vi "GCSArray_intersection.vi"(0 "Input keyword array":string[](array[string]), 1 "Available keyword array":string[](array[string]), 5 "error in (no error)":errorcluster) -> (14 "Intersection indices":i32[](array[numeric]), 19 "error out":errorcluster)   [LabVIEW 2020]
doc: "Find Intersection indices of the Input array in the Key array. The Key array acts as the master, where each element of Input array is searched. Only when equal elements are found the corresponding Input array index is added to the Intersection indices array."
panel:
  # "Find differences between two keyword arrays. Each entry of the\n'Input keyword array' is checked against any element stored in\n'Available keyword array' which acts as the master. Everytime\nan element was found its index of 'Input keyword array' is\nappended in the 'Intersection indices' list."
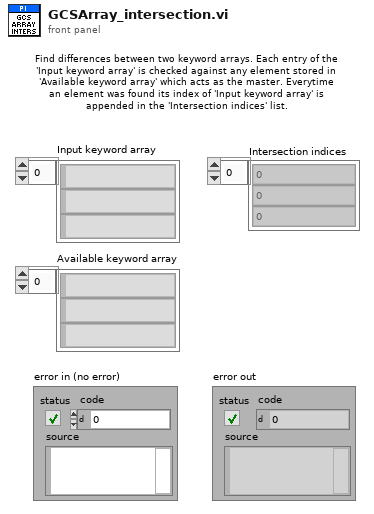
[diagram p1: front panel]
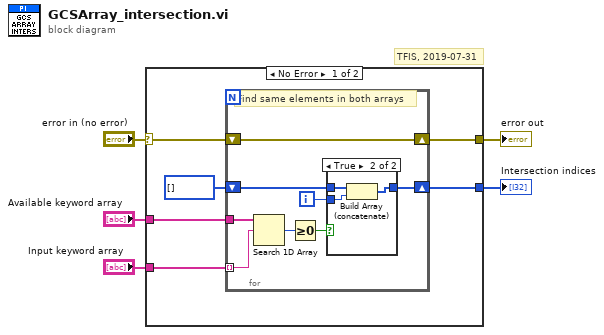
[diagram p0: block diagram]
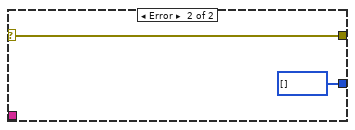
[diagram p3: hidden frame]
diagram:
  # "TFIS, 2019-07-31"
  n1 = case shown="No Error" "error in (no error)" {
    selector: "error in (no error)" -> [w11 w25]
    tunnel: [w10 w25] -> w4
    tunnel: [w9 i32[] []] -> w3
    tunnel: "Input keyword array" -> [w8 _]
    tunnel: "Available keyword array" -> [w7 _]
    frame No Error {
      n2 = for {
        tunnel: w8 -> [w18] mode=indexing
        shift-right: [w17] -> w10
        shift-left: w11 -> [w17]
        tunnel: w7 -> [w14]
        shift-right: [w12] -> w9
        shift-left: i32[] [] ("Array") -> [w13]
        i -> [w16]
        # "Find same elements in both arrays"
        n3 = Search 1D Array(1D array=w14, element=w18) -> (index of element=w19:i32)  [unwired: 1 out]
        n4 = Greater Or Equal To 0?(x=w19) -> (x >= 0?=w15:bool)
        n5 = case shown="True" w15 {
          tunnel: w13 -> [w20 w22]
          tunnel: w16 -> [_ w21]
          tunnel: [w20 w23] -> w12
          frame False {
          }
          frame True {
            n6 = Build Array (concatenate)(w22, w21) -> (w23:i32[])
          }
        }
      }
    }
    frame Error {
    }
  }
  "error out" <- w4
  "Intersection indices" <- w3
